vi "Test-All.vi"() -> ()   [LabVIEW 2023]
doc: "This VI implements the framework and scheduler for your robotics program. It should not be necessary to modify the framework. You are expected to add your code to the VIs called from Robot Main - the ones located in the Team Code folder within the project."
uses:
  <vilib>/Rock Robotics/WPI/DriverStation/WPI_DriverStationRobotMode2.ctl
  Toaster/EminemStatesEnum.ctl
  <vilib>/Rock Robotics/WPI/Simulation/Protocol/Devices/DriverStation/DS Update Ops.ctl
  <vilib>/Rock Robotics/WPI/ThirdParty/JAS_Junk/TrajLib/VI/BoolCmd_Recv.vi
  <vilib>/Rock Robotics/WPI/ThirdParty/JAS_Junk/TrajLib/VI/BoolCmd_Multiplexor_Array.vi
  Intake/IntakeStateMachine.vi
  <vilib>/Rock Robotics/WPI/ThirdParty/JAS_Junk/TrajLib/VI/DigSeqLogic_Edge_On.vi
  <vilib>/Rock Robotics/WPI/ThirdParty/JAS_Junk/TrajLib/VI/BoolCmd_Recv_Internal.vi
  <vilib>/Rock Robotics/WPI/ThirdParty/JAS_Junk/TrajLib/VI/BoolCmd_ObtainQueue.vi
  Robot Global Data.vi
  Toaster/EminemCmdPreRev.vi
  Toaster/EminemCmdShoot.vi
  Toaster/EminemCmdCancel.vi
  Toaster/EminemCmdAmp.vi
  Intake/IntakeGlobal.vi
panel:
  in  "CmdIntake":bool
  in  "CmdSpitOut":bool
  in  "CmdInc":bool
  in  "CmdDec":bool
  in  "CmdRest":bool
  in  "CmdAmp":bool
  in  "CmdSpeaker":bool
  in  "CmdCalcSpeaker":bool
  out "Low Limit Switch":bool
  out "PosDeg":dbl format="%9.1f"
  out "Shoulder MotorOutDmd":dbl format="%9.2f"
  out "IntakeMtrOut":dbl
  in  "HaveNoteSensor":bool
  out "MNM State":T1=enum."13-AmpDone"
  in  "CmdShoot":bool
  in  "CmdAmpDeliver":bool
  in  "CmdPreRev":bool
  in  "CmdCancel":bool
  out "MotorRPM Feed":dbl format="%#10.0f"
  out "MotorRPM Bot":dbl format="%#10.0f"
  out "MotorRPM Top":dbl format="%#10.0f"
  out "Robot Mode":T2
  in  "Finish":bool
  # "Amy / All"
  # "Sensor Simulation"
  # "MNM"
  # "INTAKE"
  # "SHOULDER"
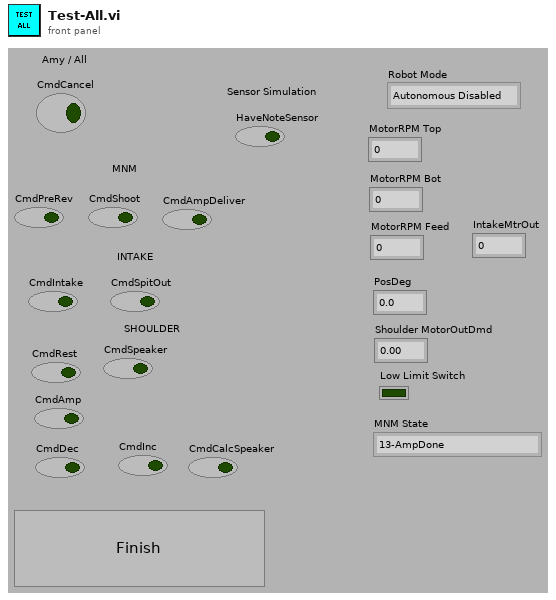
[diagram p1: front panel]
types:
  T1 = typedef "EminemStatesEnum.ctl" = enum16{"0-Init", "1-WaitForCmd", "2-Cancel", "3-ShootStart", "4-ShootRev", "5-RevUpStart", "6-ShootStartFeed&Timer", "7-ShootTimerOrSensorDone", "8-ShootDone", "9-AmpStart", "10-AmpUpToSpd?", "11-AmpStartFeed&Timer", "12-AmpTimerOrSensorDone", "13-AmpDone", "14-RevUpGetCmd"}
  T2 = typedef "WPI_DriverStationRobotMode2.ctl" = enum16{"Autonomous Disabled", "Autonomous Enabled", "Teleop Disabled", "Teleop Enabled", "Disconnected", "Finish", "Test Disabled", "Test Enabled", "Emergency Stopped"}
  T3 = typedef "WPI_DriverStationMatch Info.ctl" = cluster{"Autonomous Elapsed Seconds":dbl, "TeleOp Elapsed Seconds":dbl, "Disabled Elapsed Seconds":dbl, "Visited Autonomous":bool, "Visited TeleOp":bool, "Visited Disabled":bool, "Autonomous Settings":cluster{"Autonomous Style":enum16{"Iterative", "Independent"}, "VI Refnum":refnum<vi>}}
  T4 = typedef "WPI_DriverStationDerivedRobotMode.ctl" = enum16{"Init", "Execute", "Stop"}
  T5 = typedef "DS Update Ops.ctl" = enum16{"set enabled", "set autonomous", "set test", "set estop", "set fms", "set ds", "set control word", "set match_time", "set station", "set game data", "JSON update", "set name", "get", "transmit initial", "reset"}
  T6 = typedef "NetComm_ControlWord.ctl" = cluster{"Enabled":bool, "Autonomous":bool, "Test":bool, "E-Stop":bool, "FMS Attached":bool, "DS Attached":bool}
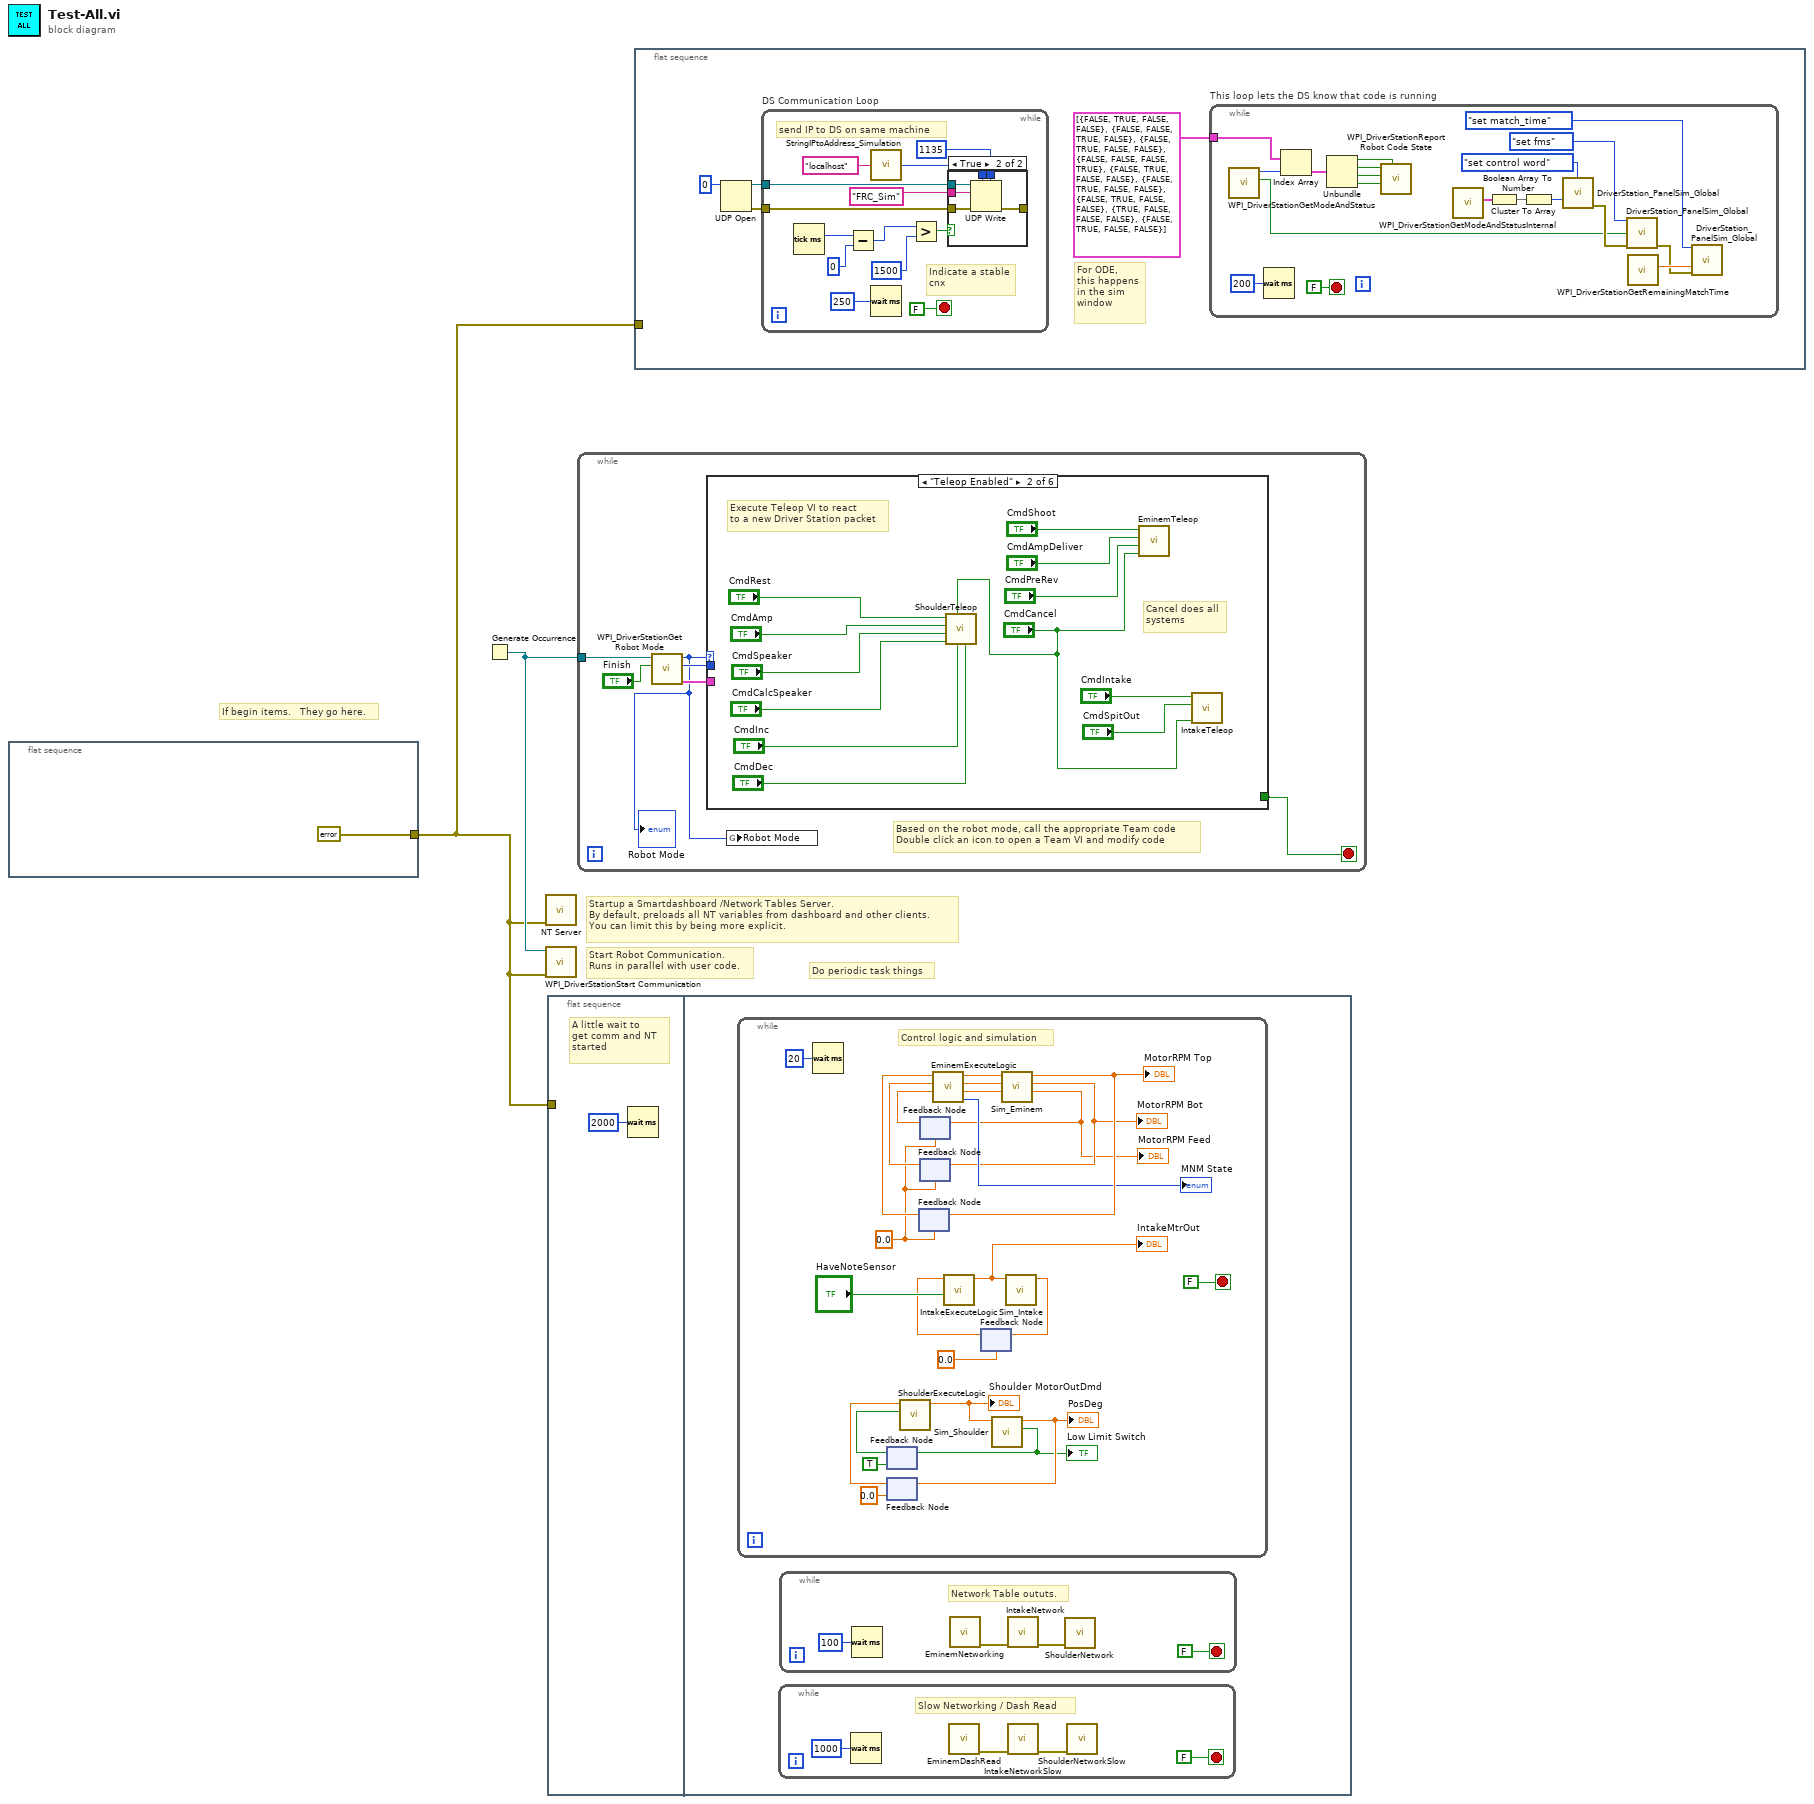
[diagram p0: block diagram]
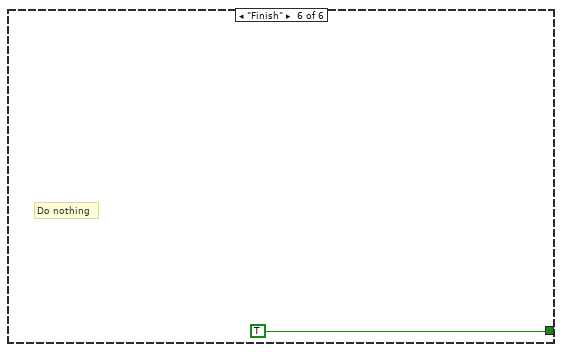
[diagram p6: hidden frame]
diagram:
  # "If begin items.   They go here."
  # "Do periodic task things"
  # "Startup a Smartdashboard /Network Tables Server.\nBy default, preloads all NT variables from dashboard and other clients.\nYou can limit this by being more explicit."
  # "Start Robot Communication.\nRuns in parallel with user code."
  n1 = flat-sequence {
    tunnel: [errorcluster {"status"=FALSE, "code"=0, "source"=""} ("error in (no error)")] -> w1
    frame #0 {
    }
  }
  n2 = Generate Occurrence() -> (w2:refnum<k4>)
  n3 = call <vilib>:"NT Server.vi"("error in (no error)"=w1) -> ()  [unwired: 10 in, 1 out]
  n4 = call <vilib>:"WPI_DriverStationStart Communication.vi"("error in (no error)"=w1, "occurrence"=w2) -> ()  [unwired: 1 in, 9 out]
  n5 = flat-sequence {
    tunnel: w1 -> [_]
    frame #0 {
      # "A little wait to\nget comm and NT\nstarted"
      n6 = Wait (ms)(milliseconds to wait=u32 2000) -> ()  [unwired: 1 out]
    }
    frame #1 {
      n7 = while {
        stop <- FALSE stop-if-true
        w27 = 0.0 ("ArmPosDeg")
        # "Control logic and simulation"
        n8 = Wait (ms)(milliseconds to wait=u32 20) -> ()  [unwired: 1 out]
        n9 = feedback #1(TRUE ("Low Limit Switch")) -> (w15:bool)
        n10 = feedback #2(0.0 ("ArmPosDeg")) -> (w17:dbl)
        n11 = call "ShoulderExecuteLogic.vi"("LowLimitSwitch"=w15, "PositionDeg"=w17) -> ("MotorDemand"=w19:dbl)  [unwired: 8 in, 1 out]
        "Shoulder MotorOutDmd" <- w19
        n12 = feedback #3(w27) -> (w33:dbl)
        n13 = feedback #4(w27) -> (w26:dbl)
        n14 = feedback #5(w27) -> (w32:dbl)
        n15 = call "EminemExecuteLogic.vi"("Feed_Vel_RPM"=w26, "Shooter_Bottom_Vel_RPM"=w32, "Shooter_Top_Vel_RPM"=w33) -> ("Box states"=→"MNM State":T1, "Shooter_Feed_Motor_Out"=w30:dbl, "Shooter_Bottom_Motor_Out"=w31:dbl, "Shooter_Top_Motor_Out"=w35:dbl)  [unwired: 5 in]
        n16 = feedback #6(0.0 ("ArmPosDeg")) -> (w20:dbl)
        n17 = call "IntakeExecuteLogic.vi"("HaveNoteSensor"="HaveNoteSensor", "Sensor Velocity"=w20) -> ("MotorOutDmd"=w23:dbl)  [unwired: 9 in]
        "IntakeMtrOut" <- w23
        n18 = call "Sim_Shoulder.vi"("Motor Dmd"=w19) -> ("Low Limit Switch"=w16:bool, "ArmPosDeg"=w18:dbl)  [unwired: 8 in, 1 out]
        "PosDeg" <- w18
        "Low Limit Switch" <- w16
        n19 = feedback-in #1(w16) -> ()
        n20 = feedback-in #2(w18) -> ()
        n21 = call "Sim_Eminem.vi"("Motor Dmd C"=w30, "Motor Dmd B"=w31, "Motor Dmd A"=w35) -> ("MotorRPM C"=w25:dbl, "MotorRPM B"=w28:dbl, "MotorRPM A"=w34:dbl)  [unwired: 6 in]
        "MotorRPM Top" <- w34
        "MotorRPM Bot" <- w28
        "MotorRPM Feed" <- w25
        n22 = feedback-in #3(w34) -> ()
        n23 = feedback-in #4(w25) -> ()
        n24 = feedback-in #5(w28) -> ()
        n25 = call "Sim_Intake.vi"("Motor Dmd"=w23) -> ("MotorRPM"=w21:dbl)  [unwired: 10 in]
        n26 = feedback-in #6(w21) -> ()
      }
      n27 = while {
        stop <- FALSE stop-if-true
        # "Slow Networking / Dash Read"
        n28 = Wait (ms)(milliseconds to wait=u32 1000) -> ()  [unwired: 1 out]
        n29 = call "EminemDashRead.vi"() -> ("error out"=w6:errorcluster)  [unwired: 11 in]
        n30 = call "IntakeNetworkSlow.vi"("error in (no error)"=w6) -> ("error out"=w5:errorcluster)  [unwired: 10 in]
        n31 = call "ShoulderNetworkSlow.vi"("error in (no error)"=w5) -> ()  [unwired: 10 in, 1 out]
      }
      n32 = while {
        stop <- FALSE stop-if-true
        # "Network Table oututs."
        n33 = Wait (ms)(milliseconds to wait=u32 100) -> ()  [unwired: 1 out]
        n34 = call "EminemNetworking.vi"() -> ("error out"=w10:errorcluster)  [unwired: 11 in]
        n35 = call "IntakeNetwork.vi"("error in (no error)"=w10) -> ("error out"=w9:errorcluster)  [unwired: 10 in]
        n36 = call "ShoulderNetwork.vi"("error in (no error)"=w9) -> ()  [unwired: 10 in, 1 out]
      }
    }
  }
  n37 = while {
    tunnel: w2 -> [w43]
    stop <- w38 stop-if-true
    # "Based on the robot mode, call the appropriate Team code\nDouble click an icon to open a Team VI and modify code"
    n38 = call <vilib>:"WPI_DriverStationGet Robot Mode.vi"("Finish"="Finish", "DS Occurrence"=w43) -> ("Match Info out"=w40:T3, "Call Context"=w42:T4, "Robot Mode"=w39:T2)  [unwired: 7 out]
    "Robot Mode" <- w39
    n39 = case shown="\"Teleop Enabled\"" w39 {
      tunnel: w42 -> [_ _ _ _ _ _]
      tunnel: w40 -> [_ _ _ _ _ _]
      tunnel: [_ _ _ _ _ TRUE] -> w38
      frame "Autonomous Enabled" {
        # "Do nothing...."
      }
      frame "Teleop Enabled" {
        # "Cancel does all\nsystems"
        # "Execute Teleop VI to react\nto a new Driver Station packet"
        n40 = call "ShoulderTeleop.vi"("CmdDownDec"="CmdDec", "CmdUpInc"="CmdInc", "CmdStop"="CmdCancel", "CmdCalcSpeaker"="CmdCalcSpeaker", "CmdSpeaker"="CmdSpeaker", "CmdAmp"="CmdAmp", "CmdRest"="CmdRest") -> ()  [unwired: 5 in]
        n41 = call "EminemTeleop.vi"("CmdCancel"="CmdCancel", "CmdPreRev"="CmdPreRev", "CmdAmpDeliver"="CmdAmpDeliver", "CmdShoot"="CmdShoot") -> ()  [unwired: 8 in]
        n42 = call "IntakeTeleop.vi"("CmdCancel"="CmdCancel", "CmdSpitOut"="CmdSpitOut", "CmdIntake"="CmdIntake") -> ()  [unwired: 9 in]
      }
      frame "Test Disabled", "Test Enabled" {
        # "Do nothing"
      }
      frame "Autonomous Disabled", "Teleop Disabled" {
        # "Do nothing."
      }
      frame "Disconnected", Default {
        # "Driver Station packet didn't arrive.\nPossibly useful for diagnostics"
      }
      frame "Finish" {
        # "Do nothing"
      }
    }
    n43 = global write "Robot Global Data.vi" "Robot Mode"(w39) -> ()
  }
  n44 = flat-sequence {
    tunnel: w1 -> [_]
    frame #0 {
      # "For ODE,\nthis happens\nin the sim\nwindow"
      n45 = UDP Open(11:u16 0 ("port")) -> (port=w60:refnum<k16>, 0:w59:errorcluster)  [unwired: 4 in, 1 out]
      n46 = while "DS Communication Loop" {
        tunnel: w60 -> [w91]
        tunnel: w59 -> [w92]
        stop <- FALSE stop-if-true
        # "Indicate a stable\ncnx"
        # "send IP to DS on same machine"
        n47 = Tick Count (ms)() -> (millisecond timer value=w81:u32)
        n48 = Subtract(x=w81, y=u32 0) -> (x-y=w84:u32)
        n49 = call <vilib>:"StringIPtoAddress_Simulation.vi"("string IP"="localhost" ("DS IP 2")) -> ("address"=w88:u32)  [unwired: 14 in]
        n50 = Wait (ms)(milliseconds to wait=u32 250) -> ()  [unwired: 1 out]
        n51 = Greater?(x=w84, y=u32 1500 ("milliseconds to wait")) -> (0:w82:bool)
        n52 = case shown="True" w82 {
          tunnel: w92 -> [_ w98]
          tunnel: w91 -> [_ w97]
          tunnel: "FRC_Sim" ("data in") -> [_ w96]
          tunnel: w88 -> [_ w95]
          tunnel: [_ w94] -> _
          tunnel: u16 1135 ("port") -> [_ w93]
          frame False {
          }
          frame True {
            n53 = UDP Write(address=w95, port or service name=w93, connection ID=w97, data in=w96, 8:w98) -> (error out=w94:errorcluster)  [unwired: 1 in, 1 out]
          }
        }
      }
      n54 = while "This loop lets the DS know that code is running" {
        tunnel: cluster{bool, bool, bool, bool}[] [{FALSE, TRUE, FALSE, FALSE}, {FALSE, FALSE, TRUE, FALSE}, {FALSE, TRUE, FALSE, FALSE}, {FALSE, FALSE, FALSE, TRUE}, {FALSE, TRUE, FALSE, FALSE}, {FALSE, TRUE, FALSE, FALSE}, {FALSE, TRUE, FALSE, FALSE}, {TRUE, FALSE, FALSE, FALSE}, {FALSE, TRUE, FALSE, FALSE}] -> [w78]
        stop <- FALSE stop-if-true
        n55 = call <vilib>:"WPI_DriverStationGetModeAndStatus.vi"() -> ("FMS Attached"=w61:bool, "Robot Mode"=w72:T2)  [unwired: 10 in]
        n56 = Wait (ms)(milliseconds to wait=u32 200) -> ()  [unwired: 1 out]
        n57 = Index Array(array=w78, index=w72) -> (element=w73:cluster{bool, bool, bool, bool})
        n58 = Unbundle(w73) -> (w79:bool, w71:bool, w76:bool, w75:bool)
        n59 = call <vilib>:"WPI_DriverStationReport Robot Code State.vi"("Test"=w79, "TeleOp"=w75, "Autonomous"=w76, "Disabled"=w71) -> ()  [unwired: 7 in, 1 out]
        n60 = call <vilib>:"WPI_DriverStationGetModeAndStatusInternal.vi"() -> ("Control Word"=w69:T6)  [unwired: 10 in, 1 out]
        n61 = Cluster To Array(cluster=w69) -> (array=w68:bool[])
        n62 = Boolean Array To Number(Boolean array=w68) -> (number=w67:u32)
        n63 = call <vilib>:"DriverStation_PanelSim_Global.vi"("menu"=DS_Update_Ops."set control word", "Numeric Value"=w67) -> ("error out"=w65:errorcluster)  [unwired: 12 in, 1 out]
        n64 = call <vilib>:"DriverStation_PanelSim_Global.vi"("menu"=DS_Update_Ops."set fms", "Value Set"=w61, "error in (no error)"=w65) -> ("error out"=w62:errorcluster)  [unwired: 11 in, 1 out]
        n65 = call <vilib>:"WPI_DriverStationGetRemainingMatchTime.vi"() -> ("Match Time(s)"=w63:sgl)  [unwired: 10 in, 1 out]
        n66 = call <vilib>:"DriverStation_PanelSim_Global.vi"("menu"=DS_Update_Ops."set match_time", "Numeric Value"=w63, "error in (no error)"=w62) -> ()  [unwired: 11 in, 2 out]
      }
    }
  }
